vi "ManipDropPiece.vi"(2 "Reinit":bool) -> (0 "error out":errorcluster, 1 "Advance Trigger":bool)   [LabVIEW 2020]
doc: "This VI commands the gripper to drop the gamepiece.\n\nParameters:\nNone"
uses:
  GlobalDriverStationCommands.vi
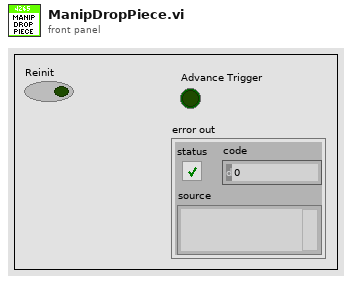
[diagram p1: front panel]
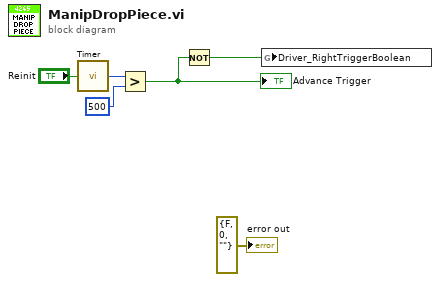
[diagram p0: block diagram]
diagram:
  n1 = call "Timer.vi"("Reset Timer"="Reinit") -> ("Time (ms)"=w5:u32)
  n2 = Greater?(x=w5, y=u32 500) -> (0:w1:bool)
  "Advance Trigger" <- w1
  n3 = Not(x=w1) -> (.not. x?=w2:bool)
  n4 = global write "GlobalDriverStationCommands.vi" "Driver_RightTriggerBoolean"(w2) -> ()
  "error out" <- errorcluster {"status"=FALSE, "code"=0, "source"=""} ("error in")
